vi "Read SCM config file.vi"(8 "Error In":errorcluster, 11 "appended path":path) -> (0 "error out":errorcluster, 1 "Array":string[](array[string]), 2 "Array 2":string[](array[string]), 3 "Refnum out":T1)   [LabVIEW 2019]
uses:
  <vilib>/Utility/config.llb/Config Data RefNum.ctl
  <vilib>/Utility/config.llb/NI_LVConfig.lvlib
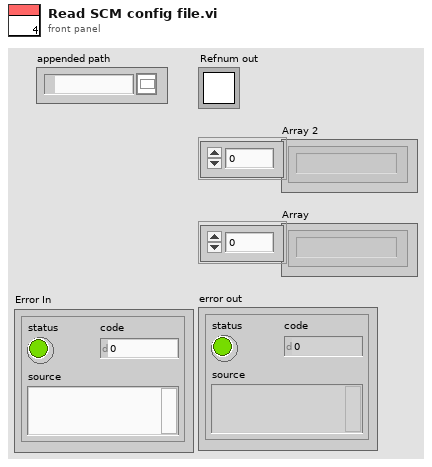
[diagram p1: front panel]
types:
  T1 = typedef "NI_LVConfig.lvlib/Config Data RefNum.ctl" = refnum<k1>
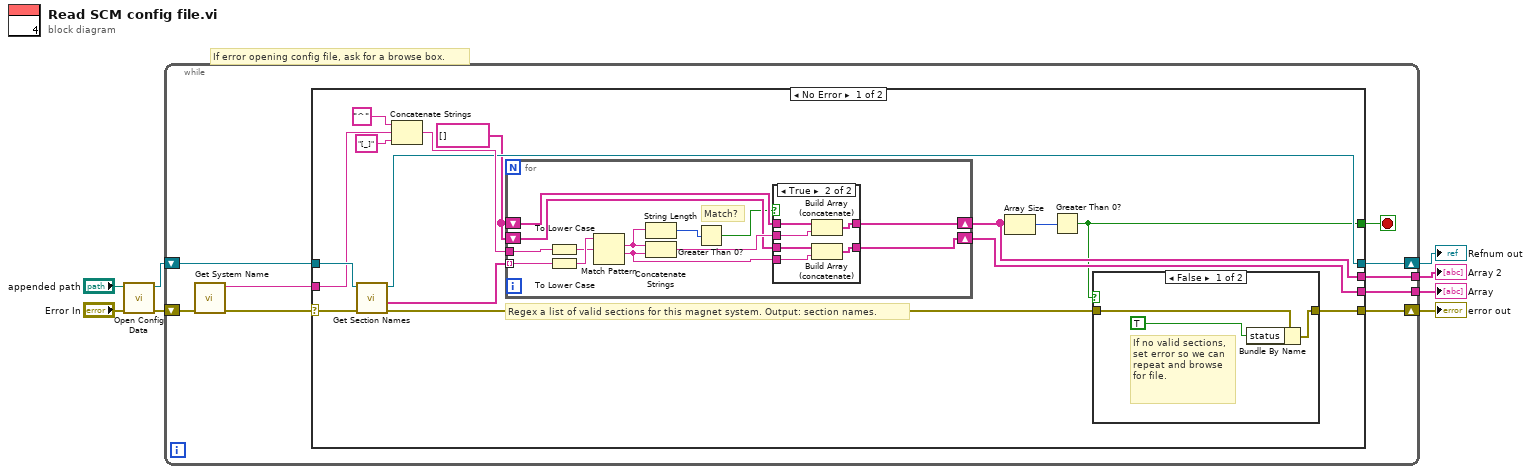
[diagram p0: block diagram]
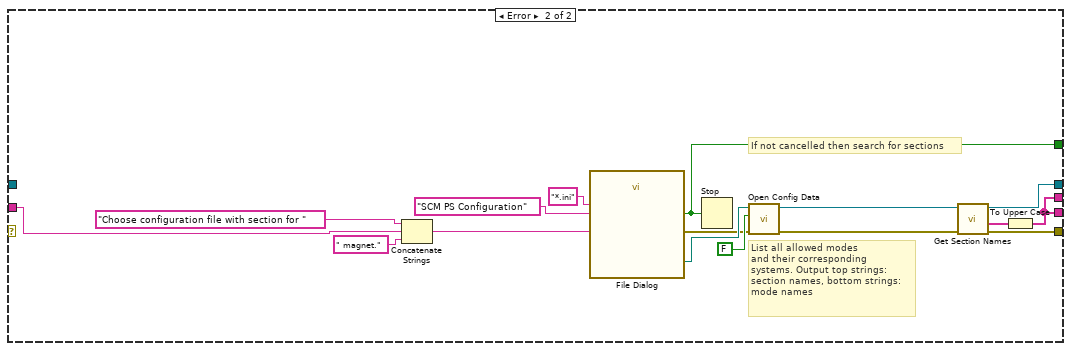
[diagram p4: hidden frame]
diagram:
  # "If error opening config file, ask for a browse box."
  n1 = call <vilib>:"Open Config Data.vi"("error in (no error)"="Error In", "configuration file path"="appended path") -> ("error out"=w6:errorcluster, "refnum"=w8:T1)  [unwired: 7 in, 1 out]
  n2 = while {
    tunnel: [w15] -> w3
    tunnel: [w13] -> w5
    shift-right: [w16] -> w2
    shift-left: w6 -> [w10]
    shift-right: [w14] -> w4
    shift-left: w8 -> [w17]
    stop <- w12 stop-if-true
    n3 = call "Get System Name.vi"("error in (no error)"=w10) -> ("error out"=w9:errorcluster, "System Name"=w11:string)  [unwired: 5 in]
    n4 = case shown="No Error" w9 {
      selector: w9 -> [w31 _]
      tunnel: w17 -> [w32 _]
      tunnel: [w19 w65] -> w16
      tunnel: [w22 w63] -> w15
      tunnel: [w26 w64] -> w14
      tunnel: [w24 w63] -> w13
      tunnel: [w21 w58] -> w12
      tunnel: w11 -> [w18 w60]
      frame No Error {
        w25 = string[] []
        # "Regex a list of valid sections for this magnet system. Output: section names."
        n5 = call <vilib>:"Get Section Names.vi"("error in (no error)"=w31, "refnum"=w32) -> ("error out"=w20:errorcluster, "section names"=w30:string[], "refnum out"=w26:T1)  [unwired: 7 in]
        n6 = Concatenate Strings("^", w18, "[_]") -> (w27:string)
        n7 = for {
          tunnel: w30 -> [w40] mode=indexing
          tunnel: w27 -> [w37]
          shift-right: [w47] -> w22
          shift-left: w25 -> [w49]
          shift-right: [w44] -> w24
          shift-left: w25 -> [w46]
          # "Match?"
          n8 = To Lower Case(string=w37) -> (all lower case string=w38:string)
          n9 = To Lower Case(string=w40) -> (all lower case string=w39:string)
          n10 = Match Pattern(string=w39, regular expression=w38) -> (match substring=w42:string, after substring=w45:string)  [unwired: 1 in, 2 out]
          n11 = String Length(string=w42) -> (length=w43:i32)
          n12 = Concatenate Strings(w42, w45) -> (w48:string)
          n13 = Greater Than 0?(x=w43) -> (x > 0?=w41:bool)
          n14 = case shown="True" w41 {
            tunnel: w49 -> [w50 w57]
            tunnel: w48 -> [_ w56]
            tunnel: [w50 w55] -> w47
            tunnel: w46 -> [w51 w54]
            tunnel: w45 -> [_ w53]
            tunnel: [w51 w52] -> w44
            frame False {
            }
            frame True {
              n15 = Build Array (concatenate)(w57, w56) -> (w55:string[])
              n16 = Build Array (concatenate)(w54, w53) -> (w52:string[])
            }
          }
        }
        n17 = Array Size(array=w22) -> (size(s)=w23:i32)
        n18 = Greater Than 0?(x=w23) -> (x > 0?=w21:bool)
        n19 = case shown="False" w21 {
          tunnel: w20 -> [w34 w36]
          tunnel: [w35 w36] -> w19
          frame False {
            # "If no valid sections, set error so we can repeat and browse for file."
            n20 = Bundle By Name(cluster=w34, "status"=TRUE) -> (w35:errorcluster)
          }
          frame True {
          }
        }
      }
      frame Error {
        # "If not cancelled then search for sections"
        # "List all allowed modes\nand their corresponding\nsystems. Output top strings: \nsection names, bottom strings:\nmode names"
        n21 = Concatenate Strings("Choose configuration file with section for " ("prompt"), w60, " magnet." ("string")) -> (w61:string)
        n22 = call "File Dialog"("prompt"=w61, "pattern (all files)"="*.ini", "pattern label"="SCM PS Configuration") -> ("selected path"=w69:path, "cancelled"=w58:bool, "error out"=w68:errorcluster)  [unwired: 9 in, 1 out]
        n23 = Stop(stop? (T)=w58) -> ()
        n24 = call <vilib>:"Open Config Data.vi"("error in (no error)"=w68, "create file if necessary (T)"=FALSE ("create file if necessary? (T)"), "configuration file path"=w69) -> ("error out"=w62:errorcluster, "refnum"=w67:T1)  [unwired: 6 in, 1 out]
        n25 = call <vilib>:"Get Section Names.vi"("error in (no error)"=w62, "refnum"=w67) -> ("error out"=w65:errorcluster, "section names"=w66:string[], "refnum out"=w64:T1)  [unwired: 7 in]
        n26 = To Upper Case(1:w66) -> (0:w63:string[])
      }
    }
  }
  "Array" <- w5
  "Refnum out" <- w4
  "Array 2" <- w3
  "error out" <- w2
